vi "Block Example.vi"(2 "Debug Mode":bool, 3 "Elapsed Time (s)":dbl, 4 "State":enum16{"Edit", "Start", "Run", "End", "Idle"}(ring), 5 "Argument List In":string[](array[string])) -> (0 "Status Out":string, 1 "Argument List Out":string[](array[string]))   [LabVIEW 2011]
doc: "This VI shows how to prevent the Growth Sequence Editor from using the \"time\" parameter for an event, and instead hand sequential control over to an API command. To do this, set the API mode to \"Continuous\" and set the options to \"Blocking\". Use the API_Unblock command in the run condition to end the API command and hand sequential control back over to the main application."
panel:
  in  "Parameter 3":dbl
  in  "Cancel":bool
  in  "Parameter 1":bool
  in  "Parameter 2":string
  in  "OK":bool
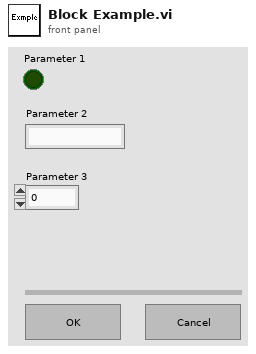
[diagram p1: front panel]
types:
  T1 = enum16{"Discrete", "Continuous", "Instantaneous"}
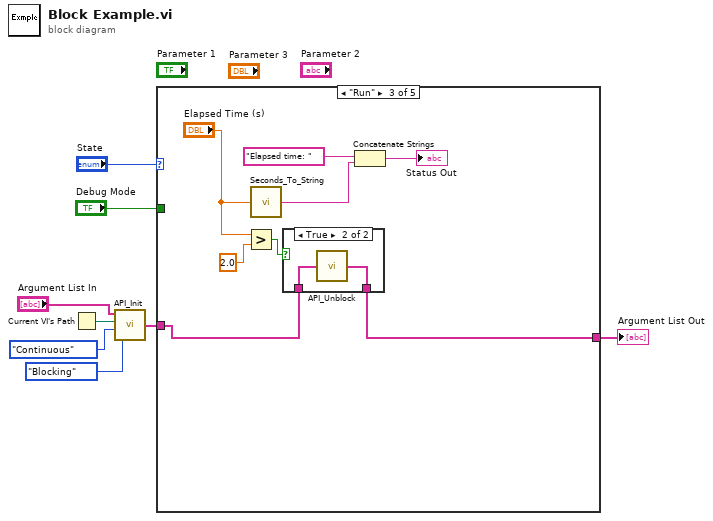
[diagram p0: block diagram]
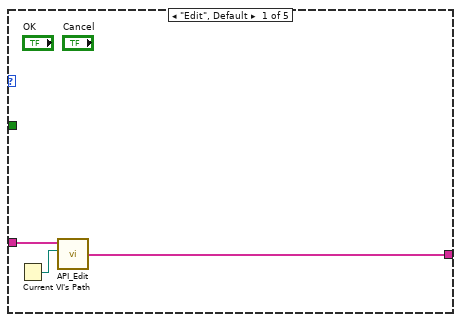
[diagram p2: hidden frame]
diagram:
  n1 = Current VI's Path() -> (path=w4:path)
  n2 = call "API_Init.vi"("API Option"=enum16{"None", "Blocking", "Wait for Input"}."Blocking", "API Mode"=T1."Continuous", "VI Path"=w4, "Argument List In"="Argument List In") -> ("Argument List Out"=w5:string[])
  n3 = case shown="\"Run\"" "State" {
    tunnel: [w9 w12 w16 w24 w25] -> w7
    tunnel: w5 -> [w11 w12 w17 w24 w25]
    tunnel: "Debug Mode" -> [_ _ _ _ _]
    frame "Edit", Default {
      n4 = Current VI's Path() -> (path=w10:path)
      n5 = call "API_Edit.vi"("VI Path"=w10, "Argument List In"=w11) -> ("Argument List Out"=w9:string[])  [unwired: 2 in]
    }
    frame "Start" {
    }
    frame "Run" {
      n6 = Greater?(x="Elapsed Time (s)", y=2.0) -> (0:w15:bool)
      n7 = call "Seconds_To_String.vi"("Seconds"="Elapsed Time (s)") -> ("Output String"=w13:string)
      n8 = case shown="True" w15 {
        tunnel: w17 -> [w21 w23]
        tunnel: [w21 w22] -> w16
        frame False {
        }
        frame True {
          n9 = call "API_Unblock.vi"("Argument List In"=w23) -> ("Argument List Out"=w22:string[])
        }
      }
      n10 = Concatenate Strings("Elapsed time: " ("string"), w13) -> (→"Status Out":string)
    }
    frame "End" {
    }
    frame "Idle" {
    }
  }
  "Argument List Out" <- w7
